vi "TablaNivelPresionSonora.vi"(8 "error in (no error)":errorcluster, 9 "fila":i32, 10 "NivelMedido":dbl, 11 "Prueba21_1 in":refnum<class "Prueba21.lvclass">) -> (0 "error out":errorcluster, 3 "Prueba21_1 out":refnum<class "Prueba21.lvclass">)   [LabVIEW 2019, in "Prueba21.lvclass"]
uses:
  Prueba21.lvclass
  Prueba21.lvclass/Prueba21.ctl
  Prueba/Prueba.lvclass
panel:
  out "array_dB":string[](array[string])
  out "array_dB (num)":dbl[](array[numeric])
  out "prom_dB":dbl
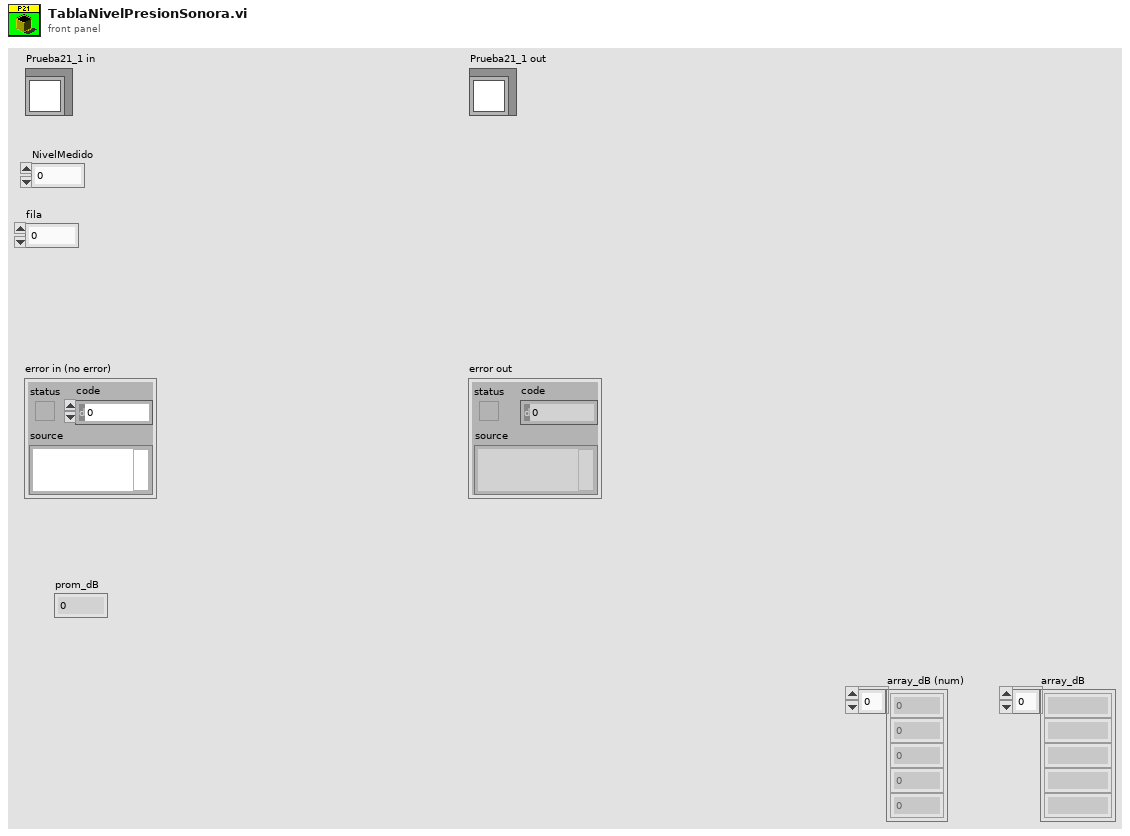
[diagram p1: front panel]
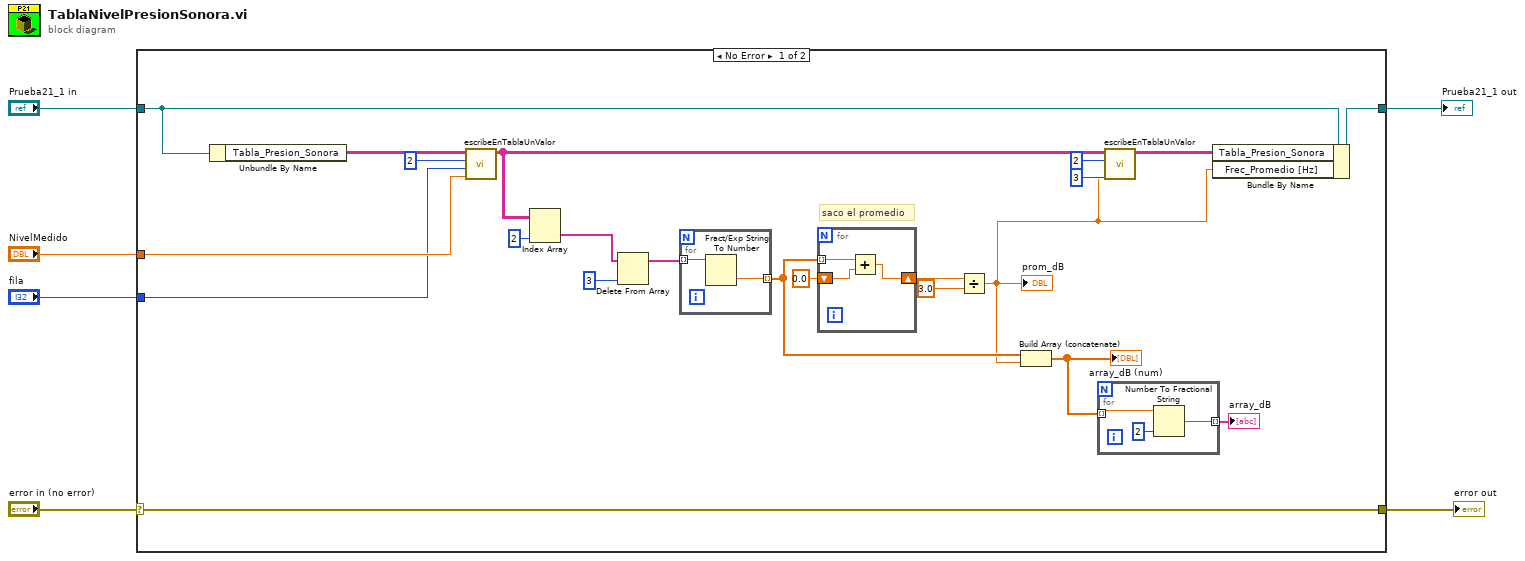
[diagram p0: block diagram]
diagram:
  n1 = case shown="No Error" "error in (no error)" {
    selector: "error in (no error)" -> [w28 w38]
    tunnel: [w28 w38] -> w5
    tunnel: [w11 w37] -> w3
    tunnel: "Prueba21_1 in" -> [w12 w37]
    tunnel: "NivelMedido" -> [w9 _]
    tunnel: "fila" -> [w8 _]
    frame No Error {
      # "saco el promedio"
      n2 = Unbundle By Name(w12) -> ("Tabla_Presion_Sonora"=w27:string[][])
      n3 = call "escribeEnTablaUnValor.vi"("element"=w9, "fila"=w8, "col"=2, "tabla in"=w27) -> ("tabla out"=w18:string[][])  [unwired: 7 in]
      n4 = Index Array "Index Array"(array=w18, index (col)=2 ("disabled index (col)")) -> (element=w21:string[])  [unwired: 1 in]
      n5 = Delete From Array(array=w21, index=3) -> (array with subset deleted=w19:string[])  [unwired: 1 in, 1 out]
      n6 = for {
        tunnel: w19 -> [w36] mode=indexing
        tunnel: [w35] -> w15 mode=indexing
        n7 = Fract/Exp String To Number(string=w36) -> (number=w35:dbl)  [unwired: 3 in, 1 out]
      }
      n8 = for {
        shift-right: [w32] -> w23
        shift-left: 0.0 ("number") -> [w33]
        tunnel: w15 -> [w34] mode=indexing
        n9 = Add(x=w34, y=w33) -> (x+y=w32:dbl)
      }
      n10 = Divide(x=w23, y=3.0) -> (x/y=w7:dbl)
      "prom_dB" <- w7
      n11 = Build Array (concatenate)(w15, w7) -> (w14:dbl[])
      "array_dB (num)" <- w14
      n12 = for {
        tunnel: w14 -> [w31] mode=indexing
        tunnel: [w29] -> w13 mode=indexing
        n13 = Number To Fractional String(number=w31, precision (6)=i16 2) -> (F-format string=w29:string)  [unwired: 2 in]
      }
      "array_dB" <- w13
      n14 = call "escribeEnTablaUnValor.vi"("element"=w7, "fila"=3, "col"=2, "tabla in"=w18) -> ("tabla out"=w10:string[][])  [unwired: 7 in]
      n15 = Bundle By Name(cluster=w12, "Tabla_Presion_Sonora"=w10, "Frec_Promedio [Hz]"=w7) -> (w11:refnum<class "Prueba21.lvclass">)
    }
    frame Error {
    }
  }
  "error out" <- w5
  "Prueba21_1 out" <- w3
